vi "Create.vi"(8 "error in (no error)":errorcluster, 9 "Broadcaster NQR":refnum<class "Message Enqueuer.lvclass">, 10 "Unregistration Msg":refnum<class "Unregistration Msg.lvclass">, 11 "Registration Msg":refnum<class "Registration Msg.lvclass">) -> (0 "error out":errorcluster, 3 "Subscription Token Out":refnum<class "Subscription Token.lvclass">)   [LabVIEW 2016, in "Data Broadcasting.lvlib" / "Subscription Token.lvclass"]
doc: "Creates a new Subscription Token. Each token carries a concrete <b>Registration Msg</b> and <b>Unregistration Msg</b> that can be sent to a specific Broadcaster using its <b>Broadcaster NQR</b> (Enqueuer).\n\n\n-------------\nCopyright (c) 2013, Staab Engineering, a Texas Limited Liability Company\nAll rights reserved.\n\nRedistribution and use in source and binary forms, with or without modification, are permitted provided that the following conditions are met:\n\n1. Redistributions of source code must retain the above copyright notice, this list of conditions and the following disclaimer.\n2. Redistributions in binary form must reproduce the above copyright notice, this list of conditions and the following disclaimer in the documentation and/or other materials provided with the distribution.\n\nTHIS SOFTWARE IS PROVIDED BY THE COPYRIGHT HOLDERS AND CONTRIBUTORS \"AS IS\" AND ANY EXPRESS OR IMPLIED WARRANTIES, INCLUDING, BUT NOT LIMITED TO, THE IMPLIED WARRANTIES OF MERCHANTABILITY AND FITNESS FOR A PARTICULAR PURPOSE ARE DISCLAIMED. IN NO EVENT SHALL THE COPYRIGHT HOLDER OR CONTRIBUTORS BE LIABLE FOR ANY DIRECT, INDIRECT, INCIDENTAL, SPECIAL, EXEMPLARY, OR CONSEQUENTIAL DAMAGES (INCLUDING, BUT NOT LIMITED TO, PROCUREMENT OF SUBSTITUTE GOODS OR SERVICES; LOSS OF USE, DATA, OR PROFITS; OR BUSINESS INTERRUPTION) HOWEVER CAUSED AND ON ANY THEORY OF LIABILITY, WHETHER IN CONTRACT, STRICT LIABILITY, OR TORT (INCLUDING NEGLIGENCE OR OTHERWISE) ARISING IN ANY WAY OUT OF THE USE OF THIS SOFTWARE, EVEN IF ADVISED OF THE POSSIBILITY OF SUCH DAMAGE."
uses:
  <userlib>/_Frameworks/Staab/AF Data Broadcasting/Data Broadcasting/Subscription Token/Subscription Token.lvclass
  <userlib>/_Frameworks/Staab/AF Data Broadcasting/Data Broadcasting/Registration Msg/Registration Msg.lvclass
  <vilib>/ActorFramework/Message Enqueuer/Message Enqueuer.lvclass
  <userlib>/_Frameworks/Staab/AF Data Broadcasting/Data Broadcasting/Unregistration Msg/Unregistration Msg.lvclass
  <userlib>/_Frameworks/Staab/AF Data Broadcasting/Data Broadcasting/Subscription Token/Subscription Token.lvclass/Subscription Token.ctl
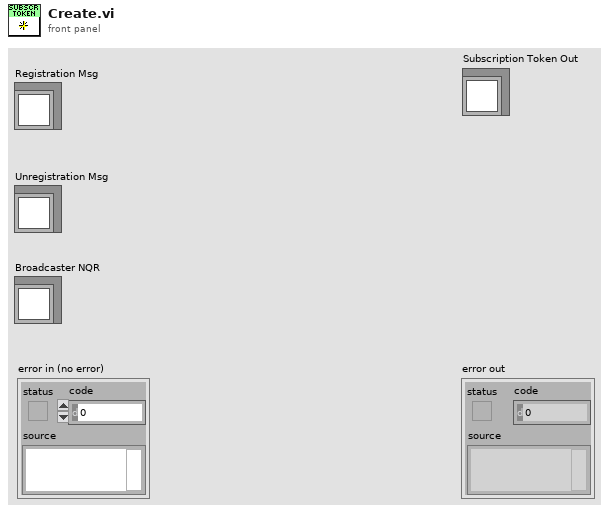
[diagram p1: front panel]
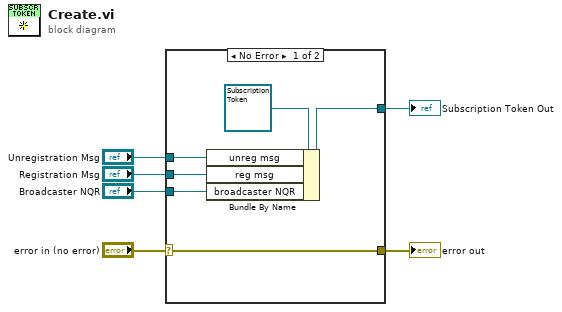
[diagram p0: block diagram]
diagram:
  n1 = case shown="No Error" "error in (no error)" {
    selector: "error in (no error)" -> [w12 w13]
    tunnel: [w12 w13] -> w5
    tunnel: [w10 _] -> w4
    tunnel: "Registration Msg" -> [w9 _]
    tunnel: "Broadcaster NQR" -> [w8 _]
    tunnel: "Unregistration Msg" -> [w7 _]
    frame No Error {
      n2 = Bundle By Name(cluster=refnum<class "Subscription Token.lvclass"> refnum ("Subscription Token in"), "unreg msg"=w7, "reg msg"=w9, "broadcaster NQR"=w8) -> (w10:refnum<class "Subscription Token.lvclass">)
    }
    frame Error {
    }
  }
  "error out" <- w5
  "Subscription Token Out" <- w4
